vi "Apply or Remove Runtime Configuration.vi"() -> ()   [LabVIEW 2026]
uses:
  <vilib>/NI VeriStand/Execution/RuntimeConfiguration/NI_VS RuntimeConfiguration ExecutionAPI.lvlib
panel:
  out "error":errorcluster
  in  "Timeout ms":u32=5000
  in  "stop":bool
  in  "Remove Configuration":bool=TRUE
  in  "Gateway IP Address (\"\": localhost)":string="localhost"
  in  "Apply Configuration":bool=TRUE
  in  "Configuration File Path":path
  in  "Runtime Configurable Section Path":string
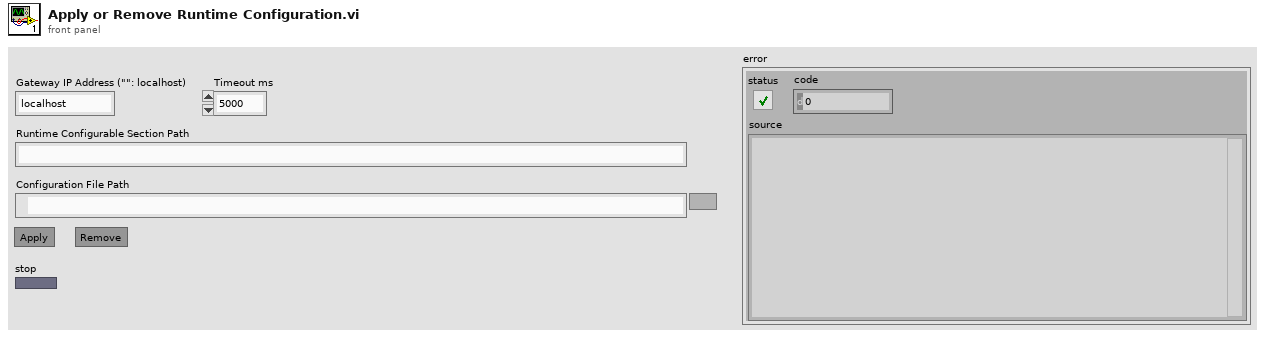
[diagram p1: front panel]
types:
  T1 = typedef "NI_VS RuntimeConfiguration ExecutionAPI.lvlib/Runtime Configuration Manager Ref.ctl" = refnum<k24>
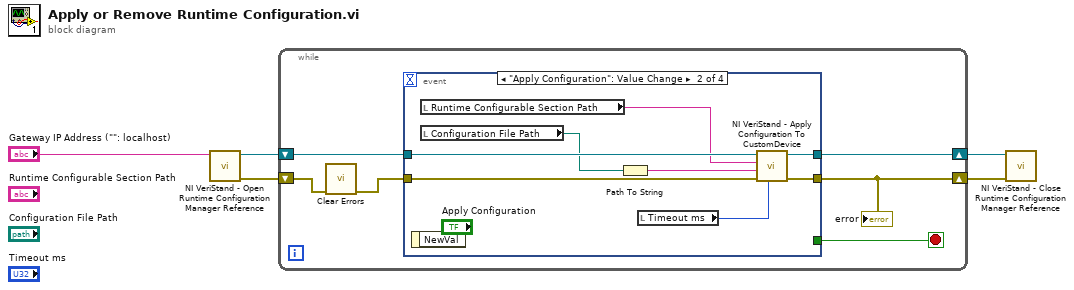
[diagram p0: block diagram]
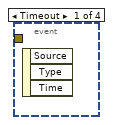
[diagram p2: hidden frame]
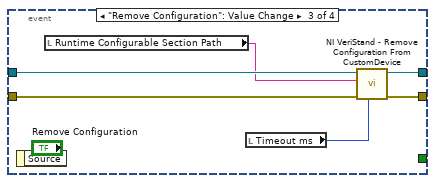
[diagram p3: hidden frame]
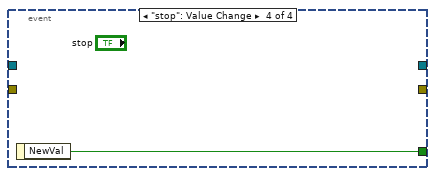
[diagram p4: hidden frame]
diagram:
  n1 = call <vilib>:"NI VeriStand - Open Runtime Configuration Manager Reference.vi"("Gateway IP Address (\"\": localhost)"="Gateway IP Address (\"\": localhost)") -> ("error out"=w5:errorcluster, "Runtime Configuration Manager"=w4:T1)  [unwired: 9 in]
  n2 = while {
    shift-right: [w9] -> w3
    shift-left: w5 -> [w7]
    shift-right: [w10] -> w2
    shift-left: w4 -> [w11]
    stop <- w8 stop-if-true
    n3 = call <vilib>:"Clear Errors.vi"("error in (no error)"=w7) -> ("error out"=w6:errorcluster)  [unwired: 5 in, 1 out]
    n4 = event shown="[1] \"Apply Configuration\": Value Change" {
      selector: _ -> [_ _ _ _]
      dyn-events: _ -> [_ _ _ _]
      timeout: _ -> [_ _ _ _]
      tunnel: w6 -> [_ w19 w23 _]
      tunnel: w11 -> [_ w18 w25 _]
      tunnel: [_ w17 w22 _] -> w9
      tunnel: [_ w16 w24 _] -> w10
      tunnel: [_ _ _ w26] -> w8
      event Timeout {
        n5 = event-data() -> ()  [unwired: 1 in, 3 out]
      }
      event "Apply Configuration": Value Change {
        n6 = event-data() -> ()  [unwired: 1 in, 1 out]
        n7 = local read "Runtime Configurable Section Path"() -> (w15:string)
        n8 = local read "Configuration File Path"() -> (w14:path)
        n9 = Path To String(path=w14) -> (string=w13:string)
        n10 = local read "Timeout ms"() -> (w12:u32)
        n11 = call <vilib>:"NI VeriStand - Apply Configuration To CustomDevice.vi"("Timeout (ms)"=w12, "error in"=w19, "Configuration File Path"=w13, "Runtime Configurable Section Path"=w15, "Runtime Configuration Manager In"=w18) -> ("error out"=w17:errorcluster, "Runtime Configuration Manager Out"=w16:T1)  [unwired: 5 in]
      }
      event "Remove Configuration": Value Change {
        n12 = event-data() -> ()  [unwired: 1 in, 1 out]
        n13 = local read "Runtime Configurable Section Path"() -> (w20:string)
        n14 = local read "Timeout ms"() -> (w21:u32)
        n15 = call <vilib>:"NI VeriStand - Remove Configuration From CustomDevice.vi"("Timeout (ms)"=w21, "error in"=w23, "Runtime Configurable Section Path"=w20, "Runtime Configuration Manager In"=w25) -> ("error out"=w22:errorcluster, "Runtime Configuration Manager Out"=w24:T1)  [unwired: 6 in]
      }
      event "stop": Value Change {
        n16 = event-data() -> ("NewVal"=w26:bool)  [unwired: 1 in]
      }
    }
    "error" <- w9
  }
  n17 = call <vilib>:"NI VeriStand - Close Runtime Configuration Manager Reference.vi"("error in"=w3, "Runtime Configuration Manager"=w2) -> ()  [unwired: 9 in, 1 out]
